vi "UnpackageMessage.vi"(10 "Message":T1) -> (1 "Value":string, 2 "Name":string)   [LabVIEW 2014, in "SimpleMessaging.lvlib"]
uses:
  SimpleMessaging.lvlib
  MessageTD.ctl
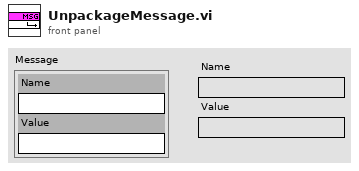
[diagram p1: front panel]
types:
  T1 = typedef "SimpleMessaging.lvlib/MessageTD.ctl" = cluster{"Name":string, "Value":string}
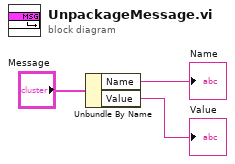
[diagram p0: block diagram]
diagram:
  n1 = Unbundle By Name("Message") -> ("Name"=→"Name":string, "Value"=→"Value":string)
